vi "macro_NumCmd_Send_TwoDbl.vi"() -> ()   [LabVIEW 2019, in "Trajectory_Library.lvlib"]
uses:
  VI/numCmd_ObtainQueue_TwoDbl.vi
  Trajectory_Library.lvlib
panel:
  in  "RightWheelDmd-Ft/Sec":dbl
  in  "LeftWheelDmd-Ft/Sec":dbl
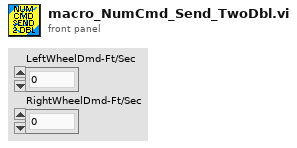
[diagram p1: front panel]
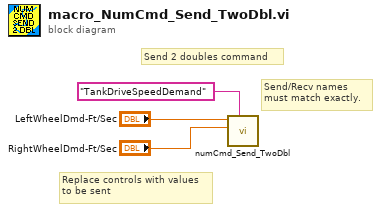
[diagram p0: block diagram]
diagram:
  # "Send/Recv names\nmust match exactly."
  # "Replace controls with values\nto be sent"
  # "Send 2 doubles command"
  n1 = call "numCmd_Send_TwoDbl.vi"("Command Name"="TankDriveSpeedDemand", "Value 2"="RightWheelDmd-Ft/Sec", "Value 1"="LeftWheelDmd-Ft/Sec") -> ()  [unwired: 8 in, 1 out]
